vi "Window-Calibration toolbox_v6.vi"() -> ()   [LabVIEW 2017]
uses:
  Configuration code/Calibration/ToolBox/TypeDefs/Current Calibration Parameters.ctl
  Configuration code/Calibration/ToolBox/TypeDefs/ProcedureState.ctl
  Typedefs/Objective selector control enum.ctl
  <vilib>/Math Plots/3D Math Plots/3D Surface/3D Surface XCtrl/3D Surface.xctl
  <vilib>/vision/Image Controls.llb/IMAQ Image.ctl
  Configuration code/Calibration/ToolBox/TypeDefs/Procedure_State.ctl
  Configuration code/Calibration/ToolBox/TypeDefs/Control Plane.ctl
  Typedefs/HW config states enum.ctl
  Peripherals Control/XYZ Stage/Typedefs/XYZ stage data.ctl
  Peripherals Control/XYZ Stage/Typedefs/XYZ stage states.ctl
  Peripherals Control/XYZ Stage/Typedefs/XYZ channel ring.ctl
  Typedefs/Top level VI states.ctl
  Global Variables/General Globals.vi
  Configuration code/Calibration/Globals/gl_Calibration globals.vi
  Global Variables/gl_UI Ctrl Refs.vi
  <vilib>/Math Plots/3D Math Plots/3D Surface/3D Surface Datatype/Public/Plot Helper (Matrix).vi
  <resource>/objmgr/IMAQImage.rc
  <vilib>/GPower/Array/GPArray.lvlib
  Global Variables/gl_Queues.vi
  <vilib>/Math Plots/3D Math Plots/3D Surface/3D Surface Datatype/3D Surface Datatype.lvclass
  <vilib>/GPower/Array/Library/Create/Random/CreateRandomI8.vi
panel:
  in  "Plot Postion":bool
  in  "Cancel Button":bool
  in  "Record Postion":bool
  in  "Z Norm":bool
  in  "Signal Channel":enum16{"Red", "Green"}(ring)
  in  "Current Objective":T1="Olympus  20X"
  out "mini steps":dbl=100.0
  out "LL":dbl=100.0 format="%#_g µm"
  out "UL":dbl=100.0 format="%#_g µm"
  in  "miniStep size":dbl=100.0 format="%#_g µm"
  in  "Sequence":bool
  in  "Test":bool
  in  "Calibrate":bool
  in  "Tab 2":T2(tab) caption="Calibration Tab"
  in  "AOLZ":sgl(slide) scale=-200.0..200.0 scale format="%#_2f"
  in  "Y Centre":sgl(slide) caption="Y centre" scale=-1.0..1.0 scale format="%#_2f"
  in  "X Centre":sgl(slide) scale=-1.0..1.0 scale format="%#_2f"
  in  "Zero Stage":bool
  in  "XY Step Size":dbl=100.0 format="%#_g µm"
  in  "Up":bool
  in  "Left":bool
  in  "Right":bool
  in  "Down":bool
  out "Focal Plane":sgl format="Z:%#_g"
  in  "Set focal plane":bool
  in  "Z Step Size":dbl=100.0 format="%#_g µm"
  in  "Natural Plane":bool
  in  "Move Down":bool
  in  "Move Up":bool
  out "Stage XYZ Position":cluster{"X":sgl, "Y":sgl, "Z":sgl}
  in  "Current Calibration Parameters":T3
  in  "Z Angle":dbl(knob)
  in  "Y Angle":dbl(knob)
  in  "X Angle":dbl(knob) min=0.0 max=359.9 step=0.1
  in  "Sweep":enum16{"Dwell Time", "SWAT"}(ring)
  in  "Multicolumn Listbox":i32(listbox)
  out "Y Scaling":cluster{"X":dbl, "Y":dbl}[](graph)
  out "X Scaling":cluster{"X":dbl, "Y":dbl}[](graph)
  out "Z Scaling":cluster{"X":dbl, "Y":dbl}[](graph)
  in  "Reload":bool
  in  "Save config.ini":bool
  out "Z plane exec time":u32
  out "3D Surface":refnum<class "3D Plot Datatype.lvclass">[](xcontrol)
  out "Intensity Graph":i16[][](graph)
  out "Image Pixels (I16)":i16[][](array[numeric])
  out "Stage Zeroed ? 2":bool
  out "AOL Z values":i32[](array[numeric])
  out "Motor Z values":i32[](array[numeric])
  out "Stage Zeroed ?":bool
  out "Z":sgl format="Z:%#_g"
  out "Y":sgl format="Y:%#_g"
  out "X":sgl format="X:%#_g"
  out "Progress":u8(slide) scale=0.0..21.0
  out "error out":errorcluster
  out "Procedure":T4
  in  "Auto Focus":bool
  in  "Message_FrontPanel":string
  in  "Cancel":bool
  in  "Abort":bool
  in  "Next":bool
  in  "N":i32=512
  out "Stop_Ind":bool
  in  "Exit":bool
  in  "Calibration Tab":T5(tab)
  in  "Live Image intensity":cluster{i16, i16}(slide)={0, 2048} scale=0.0..4095.0
  in  "Visible(Grid)":bool
  in  "Grid Lines":u32=2 min=2 max=10 step=1
  out "Image":T6(plugin-control)
  out "Array":T6[](array[plugin-control])
  out "Analysis Graph":cluster{"X":dbl, "Y":dbl}[](graph)
  out "PSF Plot":cluster{"X":dbl, "Y":dbl}[](graph)
  out "PSF Image":T6(plugin-control)
  in  "Objectives":string(tree)
  out "Calibration.ini Path":path
  out "Calibration.ini":string
  in  "Step details":string
  in  "Step No":T7(ring)
  in  "Pockels Cell Value for pointing mode":dbl
  in  "auto-set pockel":bool
  in  "Calibration_min":dbl
  in  "Calibration_max":dbl
  in  "Search_min":dbl
  in  "Search_max":dbl
  in  "Testing Range (Norm)_max":dbl=1.0
  in  "Testing Range (Norm)_min":dbl=-1.0
  in  "Auto Calibration":bool
  in  "Measure PSF":bool
  in  "Calibration test type":T8(ring)
  in  "Calibration type":T9(ring)
  # "Current XYZ Stage Position"
  # "Natural Focal Plane Z motor position must be \nset  to Zero before using the following buttons"
  # "Calibration Options"
  # "Maximal Search Range"
  # "to"
  # "(for sums &\ndiffs only)"
  # "Calibration Range from"
  # "to"
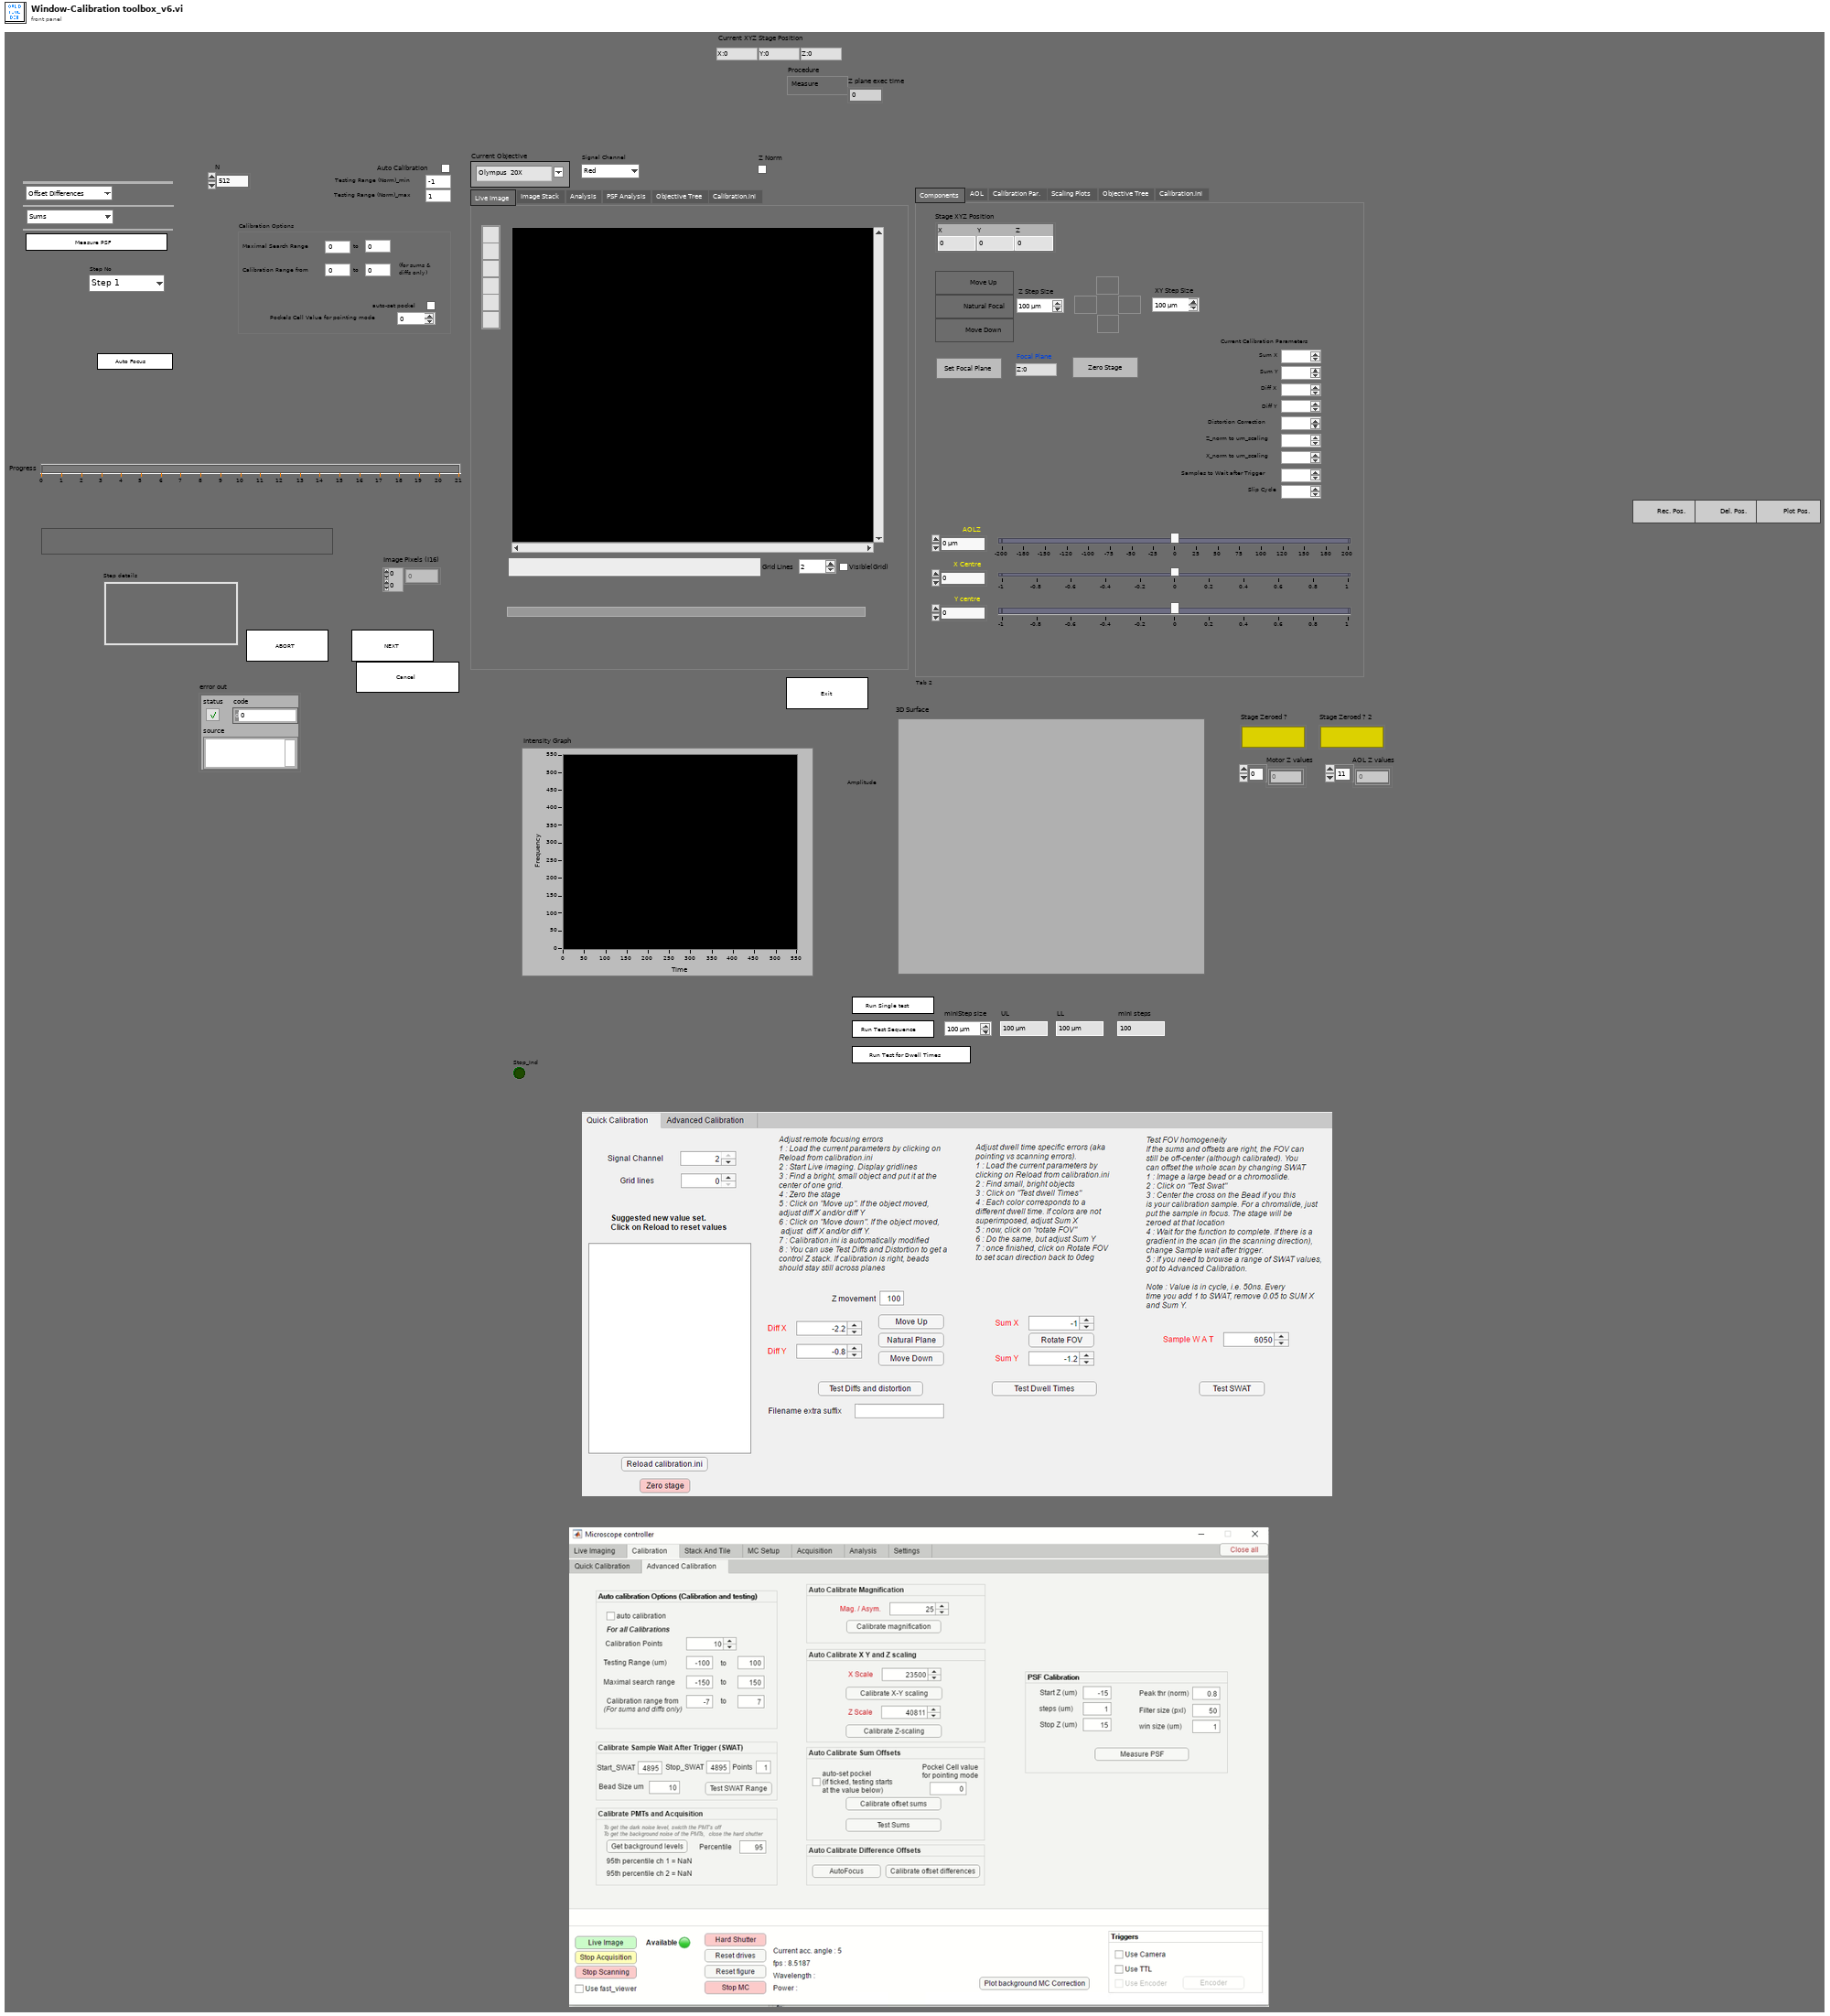
[diagram p1: front panel]
types:
  T1 = typedef "Objective selector control enum.ctl" = string
  T2 = enum32{"Components", "AOL", "Calibration Par.", "Scaling Plots", "Objective Tree", "Calibration.ini"}
  T3 = typedef "Current Calibration Parameters.ctl" = cluster{"Sum X":dbl, "Sum Y":dbl, "Diff X":dbl, "Diff Y":dbl, "Distortion Correction":dbl, "Z_norm to um_scaling":dbl, "X_norm to um_scaling":dbl, "Samples to Wait after Trigger":dbl, "Slip Cycle":dbl}
  T4 = typedef "ProcedureState.ctl" = enum16{"Measure", "Calibrate", "Sequence", "Test"}
  T5 = enum32{"Live Image", "Image Stack", "Analysis", "PSF Analysis", "Objective Tree", "Calibration.ini"}
  T6 = typedef "IMAQ Image.ctl" = refnum<image>
  T7 = enum16{"Step 1", "Step 2", "Step 3", "Step 4", "Step 5", "Step 6", "Step 7", "Step 8", "Step 9"}
  T8 = enum16{"Sums", "Diffs and Distortion", "Dwell Times"}
  T9 = enum16{"Offset Differences", "Magnification", "Offset Sums", "X-Y Scaling", "Z-Scaling"}
  T10 = enum32{"Invalid", "Standard", "Closed", "Hidden", "Minimized", "Maximized"}
  T11 = typedef "HW config states enum.ctl" = enum16{"Load from file", "Save to file", "Write all", "Read all", "Write XY stage settings", "Write DAQ FPGA settings", "Write Control FPGA settings", "Write Phys Channels", "Write System Config", "Write HW Config", "Save System Config", "Save HW Config", "Clear", "Compare from file"}
  T12 = enum8{"Enabled", "Disabled", "Disabled and Grayed Out"}
  T13 = enum16{"Initialise", "Load from file", "Save to file", "Read", "Write"}
  T14 = enum32{"Bad", "Idle", "Run top level", "Running"}
  T15 = typedef "Live graph data queue ref.ctl" = refnum<queue>
  T16 = enum32{"Image", "Image Stack", "Analysis", "PSF Analysis", "Objective Tree", "Calibration.ini"}
  T17 = typedef "Calibration config.ctl" = cluster{"Current Objective":string, "Objective Settings":T18[], "PreChirper Values Preset ?":bool, "PreChirper Settings":T19[], "PreChirper Constants":T20}
  T18 = typedef "Objective Config.ctl" = cluster{"Name":string, "Sum X":dbl, "Sum Y":dbl, "Diff X":dbl, "Diff Y":dbl, "Distortion Correction":dbl, "Z_norm to um_scaling":dbl, "X_norm to um_scaling":dbl, "Calibrated Wavelength":dbl}
  T19 = typedef "Prechirper Cal Config.ctl" = cluster{"Wavelength":i32, "Prism 1":i32, "Prism 2":i32}
  T20 = typedef "PreChirper constants.ctl" = cluster{"a 1":i32, "b 1":i32, "c 1":i32, "a 2":i32, "b 2":i32, "c 2":i32, "lmin":i32, "lmax":i32}
  T21 = typedef "System Configuration.ctl" = cluster{"Laser wavelength (nm)":dbl, "DAQ FPGA System":T22, "Control system":T23}
  T22 = typedef "DAQ FPGA system config.ctl" = cluster{"Clock Freq (MHz) ":dbl, "Samples Wait after Trigger":u16, "AOD fill":u16, "StartupDelay":i32, "Slip Cycle (clock cycles)":u32, "Add Cycle":bool}
  T23 = typedef "CTRL system config.ctl" = cluster{"AOD 1 Amplitude":i16, "AOD 2 Amplitude":i16, "AOD 3 Amplitude":i16, "AOD 4 Amplitude":i16, "AOD 5 Amplitude":i16, "AOD 6 Amplitude":i16, "T0 (ns)":dbl, "Ta (ns)":dbl, "Data Time Interval (ns)":dbl, "Ctrl FPGA Clock (MHz)":dbl}
  T24 = typedef "UI ctrl refs cluster.ctl" = cluster{"Top level VI path":path, "Top level VI ref":refnum<vi>, "User menu ref":refnum<k9>, "Sub Panel control":refnum<vi>, "Imaging Param Tab":refnum<vi>, "Occurrence-Start drivers":refnum<k4>, "Occurrence-Speed logging initialised":refnum<k4>, "Occurrence-XYZ stage initialised":refnum<k4>, "Exit button":refnum<vi>, "Status ind":refnum<vi>, "Set as origin":refnum<vi>, "Speed Logging":refnum<vi>, "Time Lapse":refnum<vi>, "Live Imaging":refnum<vi>, "AOL Z Stack":refnum<vi>, "Motor Z Stack":refnum<vi>, "Funct Acq button":refnum<vi>, "Hard Shutter":refnum<vi>, "Virtual Shutter":refnum<vi>, "Laser Power":refnum<vi>, "AOL Mode":refnum<vi>, "Frame Size":refnum<vi>, "Field of View":refnum<vi>, "Dwell Time":refnum<vi>, "Zoom":refnum<vi>, "AOL Z":refnum<vi>, "Objective":refnum<vi>, "Axis":refnum<vi>, "Paths & Names":refnum<vi>, "Experiment folder path (ind.)":refnum<vi>, "Last State (Ind.)":refnum<vi>, "Averages":refnum<vi>, "Angle (degrees)":refnum<vi>, "X centre":refnum<vi>, "Y centre":refnum<vi>, "Plane Mode":refnum<vi>, "# Planes":refnum<vi>, "Z Start":refnum<vi>, "Z Stop":refnum<vi>, "Z Step":refnum<vi>, "PMT 1":refnum<vi>, "PMT 2":refnum<vi>, "Stage XYZ Position":refnum<vi>, "Pockels@Z Start":refnum<vi>, "Pockels@Z Stop":refnum<vi>, "Obtain Z Start":refnum<vi>, "Obtain Z Stop":refnum<vi>, "Live stim.trig.period":refnum<vi>, "Live stim.trig.enable":refnum<vi>, "Movement Correction":refnum<vi>, "Load Reference Image":refnum<vi>, "XY Stage Move":refnum<vi>, "MovCor Cluster":refnum<vi>, "RefDAQParam":refnum<vi>, "Funct. Acq. Pockels Modulation":refnum<vi>, "Ref Laser Power":refnum<vi>, "Enable Video Recording":refnum<vi>, "Video Record-Live Imaging":refnum<vi>, "Video Record-Funct acq":refnum<vi>, "Reference Source":refnum<vi>, "AOL Z-stack Chirps Ready (ind)":refnum<vi>, "Target time between mov.cor. ref triggers (ms)":refnum<vi>, "Funct. Acq. Ref frame save":refnum<vi>, "Tracking button":refnum<vi>, "Show ref plots window":refnum<vi>, "Center freq ind (nm)":refnum<vi>, "Pickup mode (ind)":refnum<vi>, "Logging queue (ind)":refnum<vi>, "Back aperture power (ind.)":refnum<vi>, "Power after objective (ind.)":refnum<vi>, "Switch user":refnum<vi>, "Ls1 Conn. Status":refnum<vi>, "Ls1Tuning Status":refnum<vi>, "Ls1 Faults":refnum<vi>, "Ls1 Connection":refnum<vi>, "Ls1 Mode":refnum<vi>, "Ls1 POWER [mW]":refnum<vi>, "Ls1Shutter":refnum<vi>, "Ls1 Wavelength":refnum<vi>, "Ls1 Note":refnum<vi>, "Ls1 Confirm Wav":refnum<vi>, "Ls1 PreChrp Prism1":refnum<vi>, "Ls1 PreChrp Prism2":refnum<vi>, "Ls1 wav top Ind":refnum<vi>, "Ls1 power top Ind":refnum<vi>, "Ls1 Pump peak Hold":refnum<vi>, "Ls1 Status Ind":refnum<vi>, "Ls1 wav cancel":refnum<vi>, "Experiment Type":refnum<vi>, "Biology Information":refnum<vi>}
  T25 = typedef "AOL Z cal process refs.ctl" = cluster{"This VI":refnum<vi>, "Abort (ind)":refnum<vi>, "Next (ind)":refnum<vi>, "Cancel":refnum<vi>, "Next":refnum<vi>, "Message":refnum<vi>, "Progress":refnum<vi>}
  T26 = typedef "Image Type" = u32
  T27 = typedef "Control Plane.ctl" = enum16{"XY-X", "XY-Y", "Z"}
  T28 = typedef "Procedure_State.ctl" = cluster{"Procedure":T4, "Parameter":T27, "Symmetric":bool}
  T29 = typedef "XYZ stage states.ctl" = enum16{"Dequeue", "Initialize", "Read Position", "Read Speed Setting", "Move", "Set Max Speed", "Reset Axis", "Stop all movement"}
  T30 = typedef "XYZ channel ring.ctl" = string
  T31 = typedef "XYZ stage data.ctl" = cluster{"Command":T29, "Channel":T30, "X":sgl, "Y":sgl, "Z":sgl, "Speed":i32, "Zero":bool, "Use acknowledgement?":bool}
  T32 = typedef "Top level VI states.ctl" = enum16{"None", "Initialise UI", "<STACK PROTOCOL STATES>", "AOL Zstack-START", "AOL Zstack-STOP", "Motor Zstack-START", "Motor Zstack-STOP", "<ACQUISITION PROTOCOL STATES> ", "Functional Acquisition-START", "Functional Acquisition-STOP", "Single Plane Acquisition-START", "Single Plane Acquisition-STOP", "Volume Acquisition-START", "Volume Acquisition-STOP", "<LIVE IMAGING PROTOCOL STATES>", "Live Imaging-START", "Live Imaging-STOP", "Live Plane Imaging-START", "Live Plane Imaging-STOP", "Live Volume Imaging-START", "Live Volume Imaging-STOP", "<MOVEMENT CORRECTION PROTOCOL STATES>", "EXIT"}
  T33 = typedef "AOL_Globals.ctl" = cluster{"Imaging Protocol":T34, "Number of POI":u16, "Number of Miniscans":u16, "Number of Trials":u16, "Number of Cycles ":u64, "# Averaged Frames":u16, "Laser power (%)":u8, "Pockels (V)":dbl, "Acquisition Length (sec)":dbl, "Fill time (us)":dbl, "POI Dwell time (us)":dbl, "Miniscan Dwell time per pixel (us)":dbl, "PMT 1":dbl, "PMT 2":dbl, "Back Apperture (mA)":dbl, "Frame Size":T35, "Center Frequency":dbl, "Field of View (norm)":dbl, "DwellTime (us)":dbl, "Wavelength (nm)":dbl, "Zoom":dbl, "AOL Z":dbl, "AOL Mode":T36, "GridXY":dbl, "GridZ":dbl, "TriggerPeriod (sec)":dbl, "Number of Pixels in Miniscan":u16, "Experiment folder path":path, "X centre":dbl, "Y centre":dbl, "Angle (degrees)":dbl, "Angle Xs (degrees)":dbl, "Angle Ys (degrees)":dbl, "Plane Mode":T37, "Threshold":u16[], "Regenerate Chirps":bool, "Rectangle ROI length (pixels)":u16, "Rectangle ROI height (pixels)":u16, "AOD fill":u16, "StartupDelay":i32, "Samples Wait after Trigger":u16, "Slip Cycle":u32, "Add Cycle":bool, "Functional Mode":T38, "Z Start":dbl, "Z Stop":dbl, "# Planes":i32}
  T34 = typedef "Imaging Protocols enum.ctl" = enum16{"AOL Z-Stack", "Motor Z Stack", "Functional Acquisition", "Single Plane Acquisition", "Volume Acquisition", "Live Imaging", "Live Plane Imaging", "Live Volume Imaging"}
  T35 = typedef "Frame Size.ctl" = u16
  T36 = typedef "AOL modes.ctl" = enum16{"Raster", "Structural", "Pointing", "Mini Scan", "Alignment"}
  T37 = typedef "Plane Mode.ctl" = u16
  T38 = typedef "Functional Mode.ctl" = enum16{"Point", "Line", "Patch", "Plane", "Volume"}
  T39 = typedef "Live imaging queue element.ctl" = cluster{"Red channel":T6, "Green channel":T6, "Ref Red channel":T6, "Ref Green channel":T6, "Mov cor":bool}
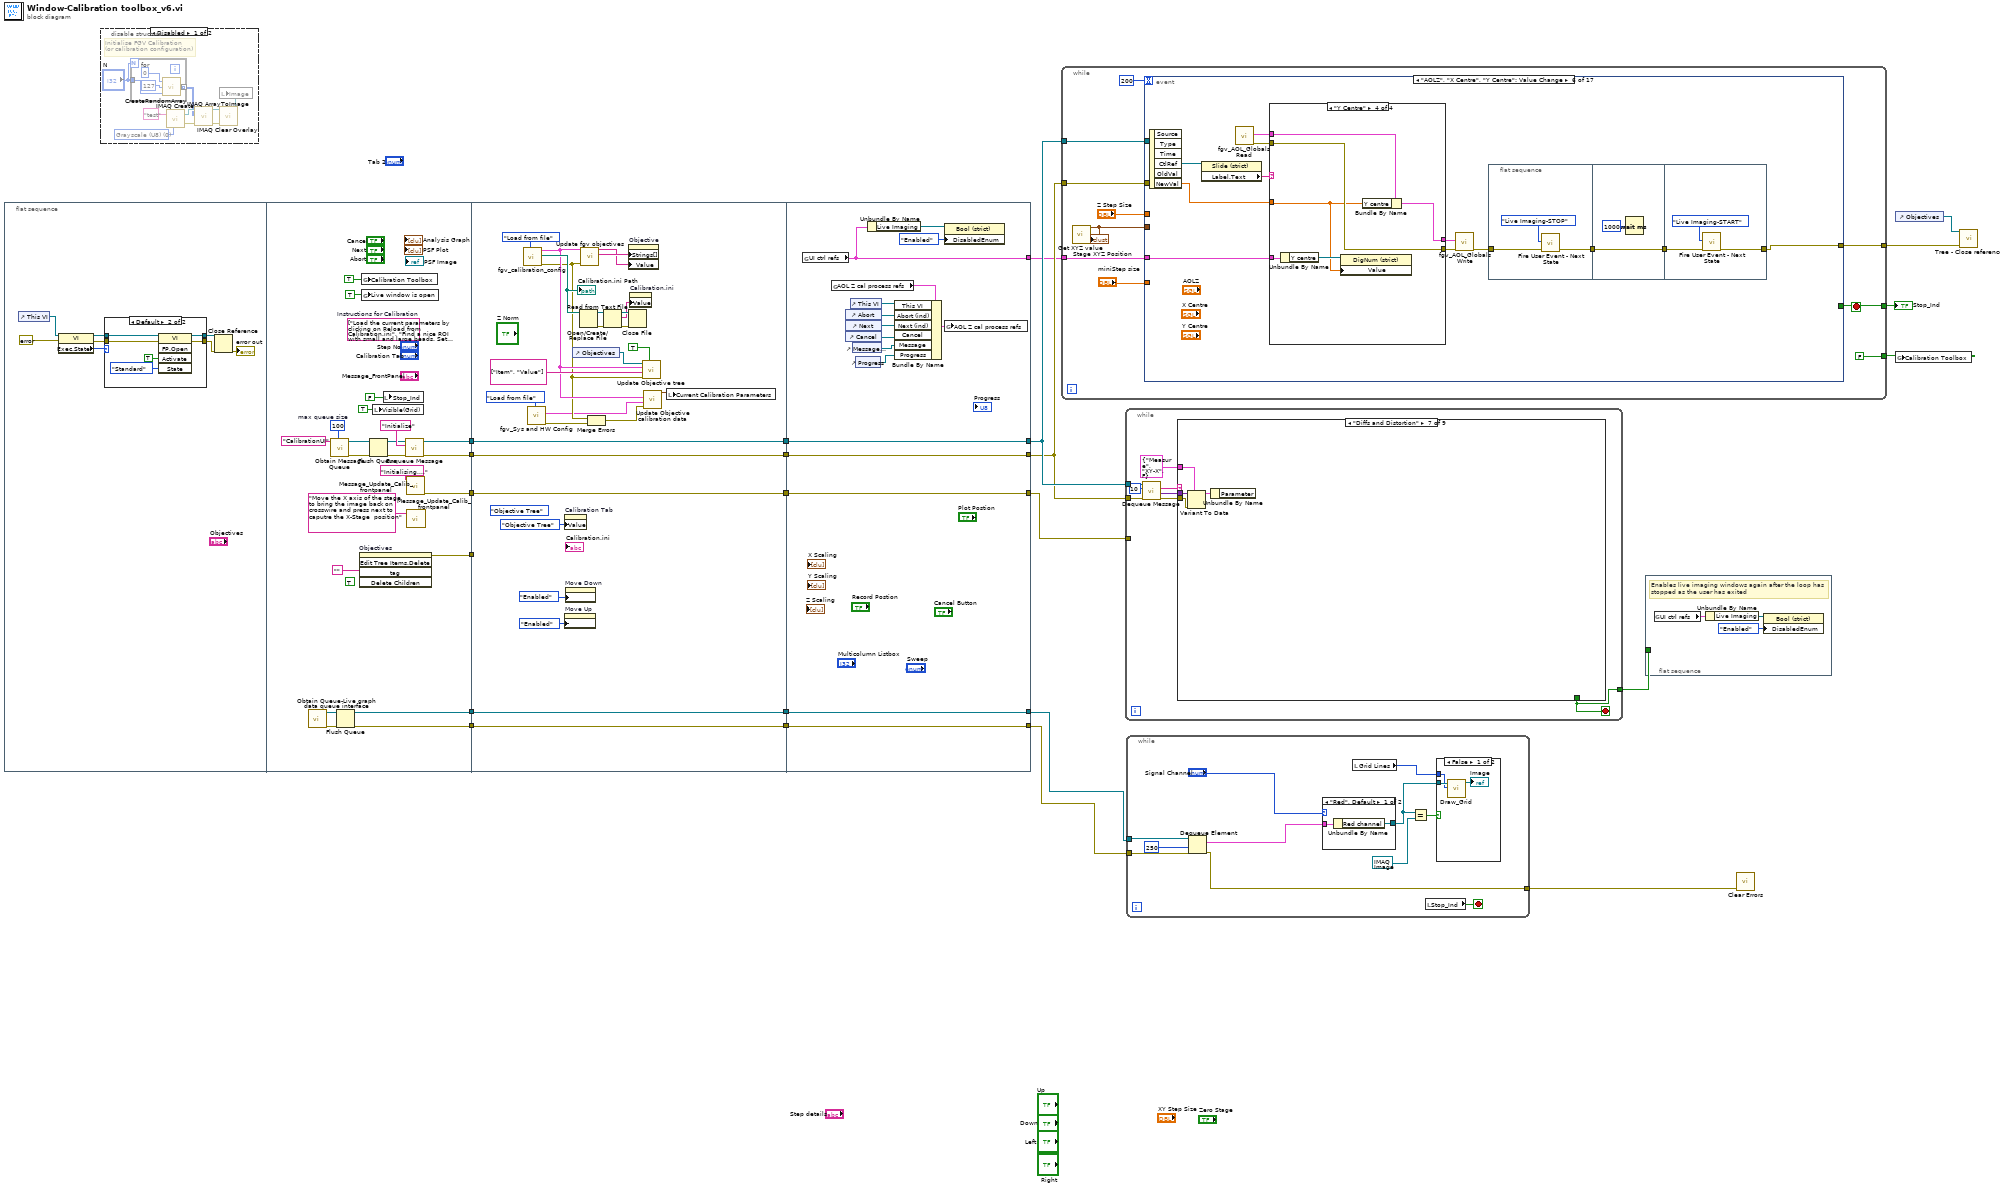
[diagram p0: block diagram]
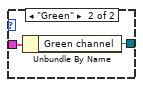
[diagram p3: hidden frame]
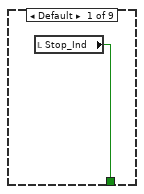
[diagram p6: hidden frame]
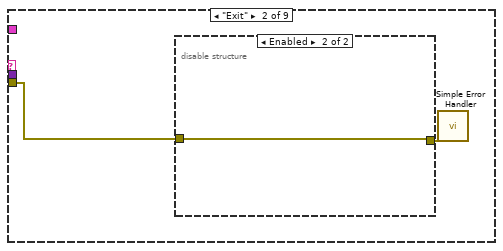
[diagram p7: hidden frame]
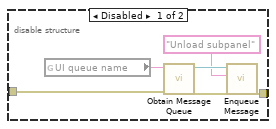
[diagram p8: hidden frame]
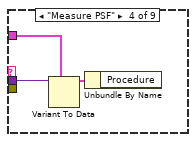
[diagram p10: hidden frame]
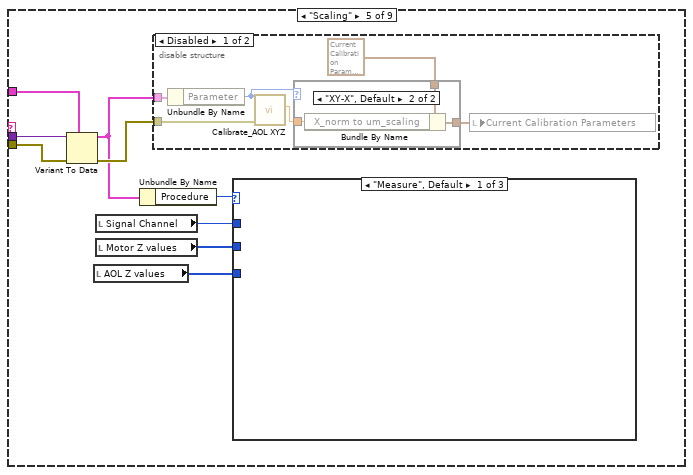
[diagram p11: hidden frame]
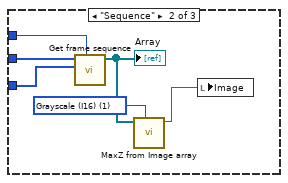
[diagram p12: hidden frame]
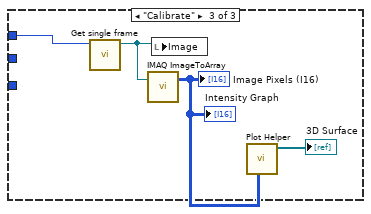
[diagram p13: hidden frame]
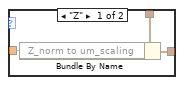
[diagram p14: hidden frame]
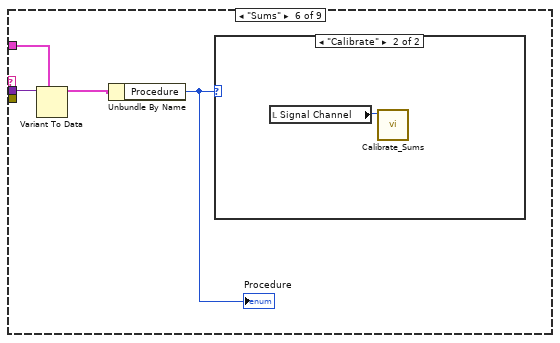
[diagram p16: hidden frame]
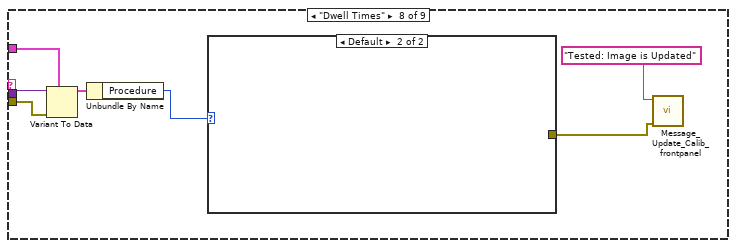
[diagram p18: hidden frame]
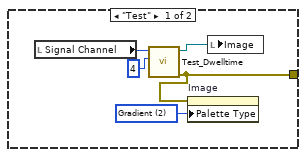
[diagram p19: hidden frame]
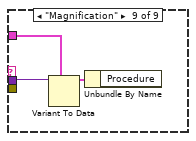
[diagram p20: hidden frame]
diagram:
  n1 = flat-sequence {
    tunnel: [w54] -> w15
    tunnel: [w53] -> w13
    tunnel: [w51] -> w11
    tunnel: [w44] -> w9
    tunnel: [w42] -> w7
    tunnel: [w41] -> w3
    tunnel: w15 -> [w88]
    tunnel: [w88] -> w14
    tunnel: w13 -> [w87]
    tunnel: [w87] -> w12
    tunnel: w11 -> [w86]
    tunnel: [w86] -> w10
    tunnel: w9 -> [w85]
    tunnel: [w85] -> w8
    tunnel: w7 -> [w84]
    tunnel: [w84] -> w6
    tunnel: w3 -> [_]
    tunnel: [w100] -> w17
    tunnel: [w101] -> w18
    tunnel: [w102] -> w19
    tunnel: [w103] -> w21
    tunnel: [w104] -> w22
    tunnel: w14 -> [w104]
    tunnel: w12 -> [w103]
    tunnel: w10 -> [w102]
    tunnel: w8 -> [w101]
    tunnel: w6 -> [w100]
    tunnel: [w92] -> w5
    frame #0 {
      n2 = control-ref of="This VI"() -> (w28:refnum<vi>)
      n3 = property class="VI"(reference=w28, error in=errorcluster {"status"=FALSE, "code"=0, "source"=""} ("error in (no error)")) -> (reference out=w27:refnum<vi>, error out=w26:errorcluster, "Exec.State"=w24:T14)
      n4 = case shown="Default" w24 {
        tunnel: [w33 w34] -> w31
        tunnel: [w32 w39] -> w30
        tunnel: w27 -> [w33 w36]
        tunnel: w26 -> [w32 w35]
        frame "Run top level" {
        }
        frame Default {
          n5 = invoke class="VI" method="FP.Open"(reference=w36, error in=w35, "Activate"=TRUE ("Activate?"), "State"=T10."Standard") -> (reference out=w34:refnum<vi>, error out=w39:errorcluster)  [unwired: 1 in, 3 out]
        }
      }
      n6 = Close Reference(reference=w31, error in (no error)=w30) -> (error out=→"error out":errorcluster)
    }
    frame #1 {
      (unwired) TRUE ("Delete Children?")
      w56 = 100  # max queue size
      (unwired) string[] ["Load the current parameters by clicking on Reload from Calibration.ini", "Find a nice ROI with small and large beads. Set PMT at 500 and adjust pockels", "Test FOV gives a sharp, single peak with Auto Focus. If yes, zero the stage. Otherwise change ROI", "Use 'Test Diffs and distortion' AND ' Test Sum' to see if the rig needs calibration for differences or sums.", "Process to teh necessary calibrations. If the performances are suboptimal, change ROI or incease laser", "If the results are bad, you can restore the previous settings by clicking on Reload from calibration.ini", "If calibration fails repetitively, try another magnification, laser pwer or FOV size.", "If calibration crashes in mid-process, go to Acquisition tab, reset drives and set the stage back to [0,0,0]. If you were in pointing mode, set teh mode toggie back to raster. Then check the pockels values."]  # Instructions for Calibration
      n7 = call "Obtain Queue-Live graph data queue interface.vi"() -> ("error out"=w45:errorcluster, "Live graphs queue"=w46:T15)  [unwired: 10 in]
      n8 = call "Obtain Message Queue.vi"("max queue size (-1, unlimited)"=w56, "Queue name"="CalibrationUI") -> ("error out"=w58:errorcluster, "Message Queue"=w60:refnum<queue>)  [unwired: 8 in]
      n9 = Flush Queue(queue=w46, error in (no error)=w45) -> (queue out=w44:T15, error out=w42:errorcluster)  [unwired: 1 out]
      n10 = invoke on="Objectives" class="Tree (strict)" method="Edit Tree Items.Delete"("tag"="") -> (error out=w41:errorcluster)  [unwired: 4 in, 4 out]
      n11 = global write "General Globals.vi" "Calibration Toolbox"(TRUE ("Calibration Toolbox")) -> ()
      n12 = global write "General Globals.vi" "Live window is open"(TRUE ("Live window is open")) -> ()
      n13 = Flush Queue(queue=w60, error in (no error)=w58) -> (queue out=w59:refnum<queue>, error out=w57:errorcluster)  [unwired: 1 out]
      n14 = local write "Visible(Grid)"(TRUE ("Visible(Grid)")) -> ()
      n15 = local write "Stop_Ind"(FALSE ("Stop_Ind")) -> ()
      n16 = call "Enqueue Message.vi"("error in (no error)"=w57, "Message"="Initialize", "Queue"=w59) -> ("error out"=w53:errorcluster, "Queue out"=w54:refnum<queue>)  [unwired: 7 in]
      n17 = call "Message_Update_Calib_frontpanel.vi"("Message"="Initialising....") -> ("error out"=w51:errorcluster)  [unwired: 10 in]
      n18 = call "Message_Update_Calib_frontpanel.vi"("Message"="Move the X axis of the stage to bring the image back on crosswire and press next to caputre the X-Stage  position") -> ()  [unwired: 10 in, 1 out]
    }
    frame #2 {
      (unwired) T16."Objective Tree" ("Calibration Tab")
      n19 = call "fgv_calibration_config.vi"("Cal config ops"=T13."Load from file") -> ("error out"=w66:errorcluster, "File Path"=w72:path, "Config cluster OUT"=w70:T17)  [unwired: 8 in]
      "Calibration.ini Path" <- w72
      n20 = call "fgv_Sys and HW Config.vi"("Function"=HW_config_states_enum."Load from file") -> ("error out"=w65:errorcluster, "System Config OUT"=w63:T21)  [unwired: 8 in, 1 out]
      n21 = property on="Calibration Tab" class="TabCtl (strict)"("Value"=T5."Objective Tree" ("Calibration Tab")) -> ()  [unwired: 2 in, 2 out]
      n22 = property on="Move Up" class="Bool"("DisabledEnum"=T12."Enabled" ("Disabled")) -> ()  [unwired: 2 in, 2 out]
      n23 = property on="Move Down" class="Bool"("DisabledEnum"=T12."Enabled" ("Disabled")) -> ()  [unwired: 2 in, 2 out]
      n24 = control-ref of="Objectives"() -> (w75:refnum<vi>)
      n25 = Open/Create/Replace File(file path (use dialog)=w72) -> (refnum out=w80:refnum<file>, error out=w79:errorcluster)  [unwired: 5 in, 1 out]
      n26 = call "Update fgv objectives.vi"("error in (no error)"=w66, "Config cluster IN"=w70) -> ("Available Objectives"=w77:string[], "Current Objective"=w76:string)  [unwired: 7 in, 1 out]
      n27 = Merge Errors(w66, w65) -> (w64:errorcluster)
      n28 = Read from Text File(file (use dialog)=w80, error in=w79) -> (refnum out=w81:refnum<file>, text=w78:string, error out=w82:errorcluster)  [unwired: 2 in, 1 out]
      n29 = property on="Objective" class="CmbBox (strict)"("Strings[]"=w77, "Value"=w76) -> ()  [unwired: 2 in, 2 out]
      n30 = Close File(refnum=w81, error in=w82) -> ()  [unwired: 2 out]
      n31 = property on="Calibration.ini" class="Str"("Value"=w78) -> ()  [unwired: 2 in, 2 out]
      n32 = call "Update Objective tree.vi"("Visible Items:Column Headers Visible"=TRUE, "error in (no error)"=w66, "Column Header Strings[]"=string[] ["Item", "Value"], "Config cluster IN"=w70, "TreeControl in"=w75) -> ()  [unwired: 6 in, 1 out]
      n33 = call "Update Objective calibration data.vi"("error in (no error)"=w64, "System Config"=w63, "Config cluster OUT"=w70) -> ("Current Calibration Parameters out"=w71:T3)  [unwired: 7 in, 1 out]
      n34 = local write "Current Calibration Parameters"(w71) -> ()
    }
    frame #3 {
      n35 = global read "gl_UI Ctrl Refs.vi" "UI ctrl refs"() -> (w92:T24)
      n36 = global read "gl_Calibration globals.vi" "AOL Z cal process refs"() -> (w94:T25)
      n37 = control-ref of="Abort"() -> (w93:refnum<vi>)
      n38 = control-ref of="Next"() -> (w99:refnum<vi>)
      n39 = control-ref of="Cancel"() -> (w95:refnum<vi>)
      n40 = control-ref of="This VI"() -> (w98:refnum<vi>)
      n41 = control-ref of="Message_FrontPanel"() -> (w96:refnum<vi>)
      n42 = control-ref of="Progress"() -> (w89:refnum<vi>)
      n43 = Unbundle By Name(w92) -> ("Live Imaging"=w91:refnum<vi>)
      n44 = Bundle By Name(cluster=w94, "This VI"=w98, "Abort (ind)"=w93, "Next (ind)"=w99, "Cancel"=w95, "Message"=w96, "Progress"=w89) -> (w97:T25)
      n45 = property class="Bool (strict)"(reference=w91, "DisabledEnum"=T12."Enabled" ("Disabled")) -> ()  [unwired: 1 in, 2 out]
      n46 = global write "gl_Calibration globals.vi" "AOL Z cal process refs"(w97) -> ()
    }
  }
  n47 = disable-structure shown="Disabled" {
    frame Disabled {
      w112 = T26 0 items=["Grayscale (U8)", "Grayscale (I16)", "Grayscale (SGL)", "Complex (CSG)", "RGB (U32)", "HSL (U32)", "RGB (U64)", "Grayscale (U16)"] ("Image Type")
      # "Initialise FGV Calibration\n(or calibration configuration)"
      n48 = for {
        N: "N" -> [_]
        tunnel: [w115] -> w109 mode=indexing
        tunnel: "N" -> [w114]
        n49 = call-poly <vilib>:"CreateRandomArray.vi"("N"=w114, "Maximum value"=i8 127, "Minimum value"=i8 0) -> ("Created array"=w115:i8[])
      }
      n50 = call "IMAQ Create"("Image Name"="test", "Image Type"=w112) -> ("New Image"=w110:T6, "error out"=w111:errorcluster)  [unwired: 3 in]
      n51 = call "IMAQ ArrayToImage"("error in (no error)"=w111, "Image Pixels (U8)"=w109, "Image"=w110) -> ("error out"=w106:errorcluster, "Image Out"=w107:T6)  [unwired: 7 in]
      n52 = call "IMAQ Clear Overlay"("error in (no error)"=w106, "Image"=w107) -> ("Image Out"=w105:T6)  [unwired: 8 in, 1 out]
      n53 = local write "Image"(w105) -> ()
    }
    frame Enabled {
    }
  }
  n54 = while {
    tunnel: [w127] -> w23
    tunnel: w22 -> [w126]
    tunnel: w21 -> [w123]
    tunnel: [FALSE ("Calibration Toolbox")] -> w20
    tunnel: w5 -> [w122]
    tunnel: [w121] -> w2
    stop <- w127 stop-if-true
    n55 = call "Get XYZ value.vi"() -> ("Stage XYZ Position"=w118:cluster{"X":sgl, "Y":sgl, "Z":sgl})  [unwired: 11 in]
    "Stage XYZ Position" <- w118
    n56 = event shown="[5] \"AOLZ\", \"X Centre\", \"Y Centre\": Value Change" {
      selector: _ -> [_ _ _ _ _ _ _ _ _ _ _ _ _ _ _ _ _]
      dyn-events: _ -> [_ _ _ _ _ _ _ _ _ _ _ _ _ _ _ _ _]
      timeout: 200 -> [_ _ _ _ _ _ _ _ _ _ _ _ _ _ _ _ _]
      tunnel: [_ TRUE _ _ _ _ _ _ _ _ _ _ _ _ _ _ _] -> w127
      tunnel: w126 -> [_ w144 _ _ _ _ _ _ w326 w380 w432 _ w455 _ _ _ _]
      tunnel: w123 -> [_ _ _ _ _ _ _ _ _ _ _ _ _ _ _ _ _]
      tunnel: w122 -> [_ _ _ w170 _ w243 w283 _ w324 w379 w422 _ _ _ _ _ _]
      tunnel: [_ _ _ _ _ w238 w278 _ _ _ _ _ _ w461 _ _ _] -> w121
      tunnel: "Z Step Size" -> [w131 _ _ w158 w237 _ _ _ _ _ _ _ _ _ _ _ _]
      tunnel: "miniStep size" -> [w130 _ _ _ w233 _ _ _ _ _ _ _ _ _ _ _ _]
      tunnel: w118 -> [w129 _ w153 w157 _ _ _ _ _ _ _ _ _ _ _ _ _]
      event Timeout {
        n57 = event-data() -> ()  [unwired: 1 in, 3 out]
        n58 = First Call?() -> (First Call?: T/F=w132:bool)
        n59 = Unbundle By Name(w129) -> ("X"=→"X":sgl, "Y"=→"Y":sgl, "Z"=w128:sgl)
        "Z" <- w128
        n60 = case shown="True" w132 {
          tunnel: w131 -> [_ w142]
          tunnel: w130 -> [_ w141]
          tunnel: w128 -> [_ w135]
          frame False {
          }
          frame True {
            n61 = Absolute Value(x=w142) -> (abs(x)=w140:dbl)
            n62 = local write "Focal Plane"(w135) -> ()
            n63 = Negate(x=w140) -> (-x=w139:dbl)
            n64 = call "Calculate Z step size.vi"("Step"=w141, "Stop"=w139, "Start"=w140) -> ("AOL Z values"=w136:dbl[], "Motor Z values"=w137:i32[], "Number of steps"=w138:i32)  [unwired: 6 in]
            n65 = local write "LL"(w139) -> ()
            n66 = local write "UL"(w140) -> ()
            n67 = local write "AOL Z values"(w136) -> ()
            n68 = local write "mini steps"(w138) -> ()
            n69 = local write "Motor Z values"(w137) -> ()
          }
        }
      }
      event Panel Close; "Exit": Value Change {
        n70 = event-data() -> ()  [unwired: 1 in, 2 out]
        n71 = case shown="True" "Exit" {
          tunnel: w144 -> [_ w151]
          frame False {
          }
          frame True {
            (unwired) enum16{"X-Y", "Z"}."X-Y" ("Parameter")
            n72 = Bundle By Name(cluster=T28 {"Procedure"=enum."Measure", "Parameter"=enum."XY-X", "Symmetric"=FALSE} ("input cluster"), "Procedure"=ProcedureState."Measure", "Parameter"=Control_Plane."XY-X") -> (w148:T28)
            n73 = call "Enqueue Message.vi"("Message Data"=w148, "Message"="Exit", "Queue"=w151) -> ()  [unwired: 7 in, 2 out]
          }
        }
      }
      event "Set focal plane": Value Change {
        n74 = event-data() -> ()  [unwired: 1 in, 6 out]
        n75 = Unbundle By Name(w153) -> ("Z"=→"Focal Plane":sgl)
      }
      event "Move Up", "Move Down", "Natural Plane": Value Change {
        n76 = event-data() -> ("CtlRef"=w173:refnum<vi>)  [unwired: 1 in, 3 out]
        n77 = Unbundle By Name(w157) -> ("Z"=w156:sgl)
        n78 = Unbundle By Name(w170) -> ("AOL Z"=w169:refnum<vi>)
        n79 = property class="Bool"(reference=w173) -> (error out=w171:errorcluster, "Label.Text"=w172:string)  [unwired: 1 in, 1 out]
        n80 = flat-sequence {
          tunnel: w172 -> [w177]
          tunnel: w171 -> [w180]
          tunnel: [w179] -> w166
          tunnel: [w178] -> w164
          tunnel: [w177] -> w162
          tunnel: [w176] -> w159
          tunnel: w158 -> [w175]
          tunnel: w156 -> [w174]
          tunnel: w166 -> [w196]
          tunnel: [w196] -> w165
          tunnel: w164 -> [w195]
          tunnel: [w195] -> w163
          tunnel: w162 -> [w194]
          tunnel: [w194] -> w161
          tunnel: [w191] -> w160
          tunnel: w159 -> [w192]
          tunnel: [w190] -> w154
          tunnel: w165 -> [w205]
          tunnel: w163 -> [w204]
          tunnel: w169 -> [w203]
          tunnel: [w202] -> w168
          tunnel: w161 -> [w202]
          tunnel: w160 -> [w201]
          tunnel: [w201] -> w167
          tunnel: [w199] -> w155
          tunnel: w154 -> [w199]
          tunnel: w168 -> [w223]
          tunnel: w167 -> [w222]
          tunnel: w155 -> [w218]
          frame #0 {
            n81 = global read "gl_Calibration globals.vi" "AOL Z cal process refs"() -> (w176:T25)
            n82 = case shown="\"Natural Plane\", Default" w177 {
              tunnel: w180 -> [_ _ _]
              tunnel: w175 -> [_ w183 w188]
              tunnel: [0.0 ("Step Size") w186 w188] -> w178
              tunnel: [w181 w184 w187] -> w179
              tunnel: w174 -> [_ w185 w189]
              frame "Natural Plane", Default {
                n83 = local read "Focal Plane"() -> (w181:sgl)
              }
              frame "Move Up" {
                n84 = Add(x=w183, y=w185) -> (x+y=w184:dbl)
                n85 = Negate(x=w183) -> (-x=w186:dbl)
              }
              frame "Move Down" {
                n86 = Subtract(x=w189, y=w188) -> (x-y=w187:dbl)
              }
            }
          }
          frame #1 {
            n87 = Unbundle By Name(w192) -> ("Message"=w191:refnum<vi>)
            n88 = disable-structure shown="Disabled" {
              frame Disabled {
                w197 = T12."Disabled and Grayed Out" ("Disabled")
                n89 = property on="Move Up" class="Bool"("DisabledEnum"=w197) -> ()  [unwired: 2 in, 2 out]
                n90 = property on="Move Down" class="Bool"("DisabledEnum"=w197) -> ()  [unwired: 2 in, 2 out]
                n91 = property on="Natural Plane" class="Bool"("DisabledEnum"=w197) -> ()  [unwired: 2 in, 2 out]
              }
              frame Enabled {
              }
            }
            n92 = property class="Str"(reference=w191, "Value"="Adjusting...") -> ()  [unwired: 1 in, 2 out]
            n93 = Tick Count (ms)() -> (millisecond timer value=w190:u32)
          }
          frame #2 {
            n94 = disable-structure shown="Enabled" {
              disable-tunnel: [w215 errorcluster {"status"=FALSE, "code"=0, "source"=""} ("error in")] -> w209
              disable-tunnel: w204 -> [w214 _]
              disable-tunnel: w203 -> [w213 _]
              frame Disabled {
                n95 = property class="Slide (strict)"(reference=w213, "Value"=w214) -> (error out=w215:errorcluster)  [unwired: 1 in, 1 out]
                n96 = call "fgv_AOL_Globals Read.vi"() -> ("AOL_Globals"=w211:T33)  [unwired: 9 in, 2 out]
                n97 = Bundle By Name(cluster=w211, "AOL Z"=w214) -> (w212:T33)
                n98 = call "fgv_AOL_Globals Write.vi"("AOL_Globals"=w212) -> ()  [unwired: 10 in, 1 out]
              }
              frame Enabled {
              }
            }
            n99 = Bundle By Name(cluster=T31 {"Command"=enum."Initialize", "Channel"="Z", "X"=0.0, "Y"=0.0, "Z"=0.0, "Speed"=0, "Zero"=FALSE, "Use acknowledgement?"=TRUE} ("XYZ Stage data to queue"), "Command"=XYZ_stage_states."Move", "Channel"=T30 "Z", "Z"=w205, "Use acknowledgement?"=FALSE) -> (w210:T31)
            n100 = call "XYZ Stage-Command request module.vi"("error in"=w209, "Command"=XYZ_stage_states."Move", "XYZ Stage data to queue"=w210) -> ()  [unwired: 4 in, 5 out]
          }
          frame #3 {
            n101 = disable-structure shown="Disabled" {
              disable-tunnel: w223 -> [w224 _]
              frame Disabled {
                n102 = case shown="\"Natural Plane\", Default" w224 {
                  frame "Move Up" {
                    n103 = property on="Move Down" class="Bool"("DisabledEnum"=T12."Enabled" ("Disabled")) -> ()  [unwired: 2 in, 2 out]
                    n104 = property on="Move Up" class="Bool"("DisabledEnum"=T12."Disabled and Grayed Out" ("Disabled")) -> ()  [unwired: 2 in, 2 out]
                  }
                  frame "Move Down" {
                    n105 = property on="Move Up" class="Bool"("DisabledEnum"=T12."Enabled" ("Disabled")) -> ()  [unwired: 2 in, 2 out]
                    n106 = property on="Move Down" class="Bool"("DisabledEnum"=T12."Disabled and Grayed Out" ("Disabled")) -> ()  [unwired: 2 in, 2 out]
                  }
                  frame "Natural Plane", Default {
                    n107 = property on="Move Up" class="Bool"("DisabledEnum"=T12."Enabled" ("Disabled")) -> ()  [unwired: 2 in, 2 out]
                    n108 = property on="Move Down" class="Bool"("DisabledEnum"=T12."Enabled" ("Disabled")) -> ()  [unwired: 2 in, 2 out]
                  }
                }
              }
              frame Enabled {
              }
            }
            n109 = Tick Count (ms)() -> (millisecond timer value=w219:u32)
            n110 = Subtract(x=w219, y=w218) -> (x-y=→"Z plane exec time":u32)
            n111 = property on="Natural Plane" class="Bool"("DisabledEnum"=T12."Enabled" ("Disabled")) -> ()  [unwired: 2 in, 2 out]
            n112 = property class="Str"(reference=w222, "Value"="Done") -> ()  [unwired: 1 in, 2 out]
          }
        }
      }
      event "Z Step Size", "miniStep size": Value Change {
        n113 = event-data() -> ()  [unwired: 1 in, 6 out]
        n114 = Absolute Value(x=w237) -> (abs(x)=w236:dbl)
        "UL" <- w236
        n115 = Negate(x=w236) -> (-x=w235:dbl)
        "LL" <- w235
        n116 = call "Calculate Z step size.vi"("Step"=w233, "Stop"=w235, "Start"=w236) -> ("AOL Z values"=→"AOL Z values":dbl[], "Motor Z values"=→"Motor Z values":i32[], "Number of steps"=→"mini steps":i32)  [unwired: 6 in]
      }
      event "AOLZ", "X Centre", "Y Centre": Value Change {
        n117 = event-data() -> ("CtlRef"=w249:refnum<vi>, "NewVal"=w242:sgl)  [unwired: 1 in, 4 out]
        n118 = property class="Slide (strict)"(reference=w249) -> ("Label.Text"=w248:string)  [unwired: 1 in, 2 out]
        n119 = call "fgv_AOL_Globals Read.vi"() -> ("error out"=w244:errorcluster, "AOL_Globals"=w247:T33)  [unwired: 9 in, 1 out]
        n120 = case shown="\"Y Centre\"" w248 {
          tunnel: w247 -> [w259 w264 w271 w277]
          tunnel: [w259 w262 w270 w275] -> w246
          tunnel: [w258 w263 w269 w276] -> w245
          tunnel: w244 -> [w258 w263 w269 w276]
          tunnel: w242 -> [_ w261 w266 w272]
          tunnel: w243 -> [_ w260 w268 w274]
          frame Default {
          }
          frame "AOLZ" {
            n121 = Unbundle By Name(w260) -> ("AOL Z"=w265:refnum<vi>)
            n122 = property class="Slide (strict)"(reference=w265, "Value"=w261) -> ()  [unwired: 1 in, 2 out]
            n123 = Bundle By Name(cluster=w264, "Y centre"=w261) -> (w262:T33)
          }
          frame "X Centre" {
            n124 = Unbundle By Name(w268) -> ("X centre"=w267:refnum<vi>)
            n125 = Bundle By Name(cluster=w271, "X centre"=w266) -> (w270:T33)
            n126 = property class="DigNum (strict)"(reference=w267, "Value"=w266) -> ()  [unwired: 1 in, 2 out]
          }
          frame "Y Centre" {
            n127 = Unbundle By Name(w274) -> ("Y centre"=w273:refnum<vi>)
            n128 = property class="DigNum (strict)"(reference=w273, "Value"=w272) -> ()  [unwired: 1 in, 2 out]
            n129 = Bundle By Name(cluster=w277, "Y centre"=w272) -> (w275:T33)
          }
        }
        n130 = call "fgv_AOL_Globals Write.vi"("error in (no error)"=w245, "AOL_Globals"=w246) -> ("error out"=w239:errorcluster)  [unwired: 9 in]
        n131 = flat-sequence {
          tunnel: w239 -> [w251]
          tunnel: [w250] -> w241
          tunnel: [w254] -> w240
          tunnel: w241 -> [w254]
          tunnel: w240 -> [w257]
          tunnel: [w256] -> w238
          frame #0 {
            n132 = call "Fire User Event - Next State.vi"("Error In"=w251, "\"UI Handler loop\" case to execute"=Top_level_VI_states."Live Imaging-STOP" ("event data / imaging mode")) -> ("Error Out"=w250:errorcluster)  [unwired: 9 in]
          }
          frame #1 {
            n133 = Wait (ms)(milliseconds to wait=u32 1000) -> ()  [unwired: 1 out]
          }
          frame #2 {
            n134 = call "Fire User Event - Next State.vi"("Error In"=w257, "\"UI Handler loop\" case to execute"=Top_level_VI_states."Live Imaging-START" ("event data / imaging mode")) -> ("Error Out"=w256:errorcluster)  [unwired: 9 in]
          }
        }
      }
      event "X Angle", "Y Angle", "Z Angle": Value Change {
        n135 = event-data() -> ("CtlRef"=w289:refnum<vi>, "NewVal"=w282:dbl)  [unwired: 1 in, 4 out]
        n136 = property class="Knob (strict)"(reference=w289) -> ("Label.Text"=w288:string)  [unwired: 1 in, 2 out]
        n137 = call "fgv_AOL_Globals Read.vi"() -> ("error out"=w287:errorcluster, "AOL_Globals"=w284:T33)  [unwired: 9 in, 1 out]
        n138 = case shown="\"Z Angle\"" w288 {
          tunnel: [w299 w300 w306 w311] -> w286
          tunnel: w287 -> [w299 w300 w306 w311]
          tunnel: [w298 w301 w305 w312] -> w285
          tunnel: w284 -> [w298 w303 w307 w313]
          tunnel: w283 -> [_ _ _ w309]
          tunnel: w282 -> [_ w302 w304 w308]
          frame Default {
          }
          frame "X Angle" {
            n139 = Bundle By Name(cluster=w303, "Angle Xs (degrees)"=w302) -> (w301:T33)
          }
          frame "Y Angle" {
            n140 = Bundle By Name(cluster=w307, "Angle Ys (degrees)"=w304) -> (w305:T33)
          }
          frame "Z Angle" {
            n141 = Unbundle By Name(w309) -> ("Angle (degrees)"=w310:refnum<vi>)
            n142 = property class="DigNum (strict)"(reference=w310, "Value"=w308) -> ()  [unwired: 1 in, 2 out]
            n143 = Bundle By Name(cluster=w313, "Angle (degrees)"=w308) -> (w312:T33)
          }
        }
        n144 = call "fgv_AOL_Globals Write.vi"("error in (no error)"=w286, "AOL_Globals"=w285) -> ("error out"=w281:errorcluster)  [unwired: 9 in]
        n145 = flat-sequence {
          tunnel: w281 -> [w291]
          tunnel: [w290] -> w279
          tunnel: [w294] -> w280
          tunnel: w279 -> [w294]
          tunnel: w280 -> [w297]
          tunnel: [w296] -> w278
          frame #0 {
            n146 = call "Fire User Event - Next State.vi"("Error In"=w291, "\"UI Handler loop\" case to execute"=Top_level_VI_states."Live Imaging-STOP" ("event data / imaging mode")) -> ("Error Out"=w290:errorcluster)  [unwired: 9 in]
          }
          frame #1 {
            n147 = Wait (ms)(milliseconds to wait=u32 100) -> ()  [unwired: 1 out]
          }
          frame #2 {
            n148 = call "Fire User Event - Next State.vi"("Error In"=w297, "\"UI Handler loop\" case to execute"=Top_level_VI_states."Live Imaging-START" ("event data / imaging mode")) -> ("Error Out"=w296:errorcluster)  [unwired: 9 in]
          }
        }
      }
      event "Save config.ini": Value Change {
        n149 = event-data() -> ()  [unwired: 1 in, 6 out]
      }
      event "Calibrate": Value Change {
        (unwired) T16."Image" ("Calibration Tab")
        n150 = event-data() -> ("NewVal"=w327:bool)  [unwired: 1 in]
        n151 = Unbundle By Name(w324) -> ("Stage XYZ Position"=w323:refnum<vi>)
        n152 = property class="Clust (strict)"(reference=w323) -> ("Value"=w322:cluster{"X":sgl, "Y":sgl, "Z":sgl})  [unwired: 1 in, 2 out]
        n153 = Unbundle By Name(w322) -> ("X"=w321:sgl, "Y"=w320:sgl, "Z"=w319:sgl)
        n154 = Equal To 0?(x=w321) -> (x = 0?=w318:bool)
        n155 = Equal To 0?(x=w320) -> (x = 0?=w317:bool)
        n156 = Equal To 0?(x=w319) -> (x = 0?=w316:bool)
        n157 = Compound Arithmetic op=AND(w318, w317, w316) -> (w315:bool)
        n158 = case shown="True" w315 {
          selector: w315 -> [_ w328]
          frame False {
          }
          frame True {
            "Stage Zeroed ?" <- w328
          }
        }
        n159 = case shown="True" w327 {
          tunnel: w326 -> [_ w331]
          tunnel: "Calibration type" -> [_ w330]
          frame False {
          }
          frame True {
            n160 = case shown="True" TRUE {
              tunnel: w331 -> [_ w340]
              tunnel: w330 -> [_ w338]
              frame False {
                n161 = One Button Dialog(message="Please move the bead to a central position and\n'zero' the XYZ stage ") -> ()  [unwired: 1 in, 1 out]
              }
              frame True {
                (unwired) enum16{"X-Y", "Z"}."X-Y" ("Parameter")
                n162 = Bundle By Name(cluster=T28 {"Procedure"=enum."Measure", "Parameter"=enum."XY-X", "Symmetric"=FALSE} ("input cluster"), "Procedure"=ProcedureState."Calibrate", "Parameter"=Control_Plane."XY-X") -> (w334:T28)
                n163 = disable-structure shown="Enabled" {
                  disable-tunnel: [w344 w368] -> w341
                  disable-tunnel: [w343 w367] -> w339
                  disable-tunnel: w338 -> [w342 _]
                  disable-tunnel: "Scaling" ("Message") -> [_ w368]
                  disable-tunnel: w334 -> [_ w367]
                  frame Disabled {
                    n164 = case shown="\"Z-Scaling\"" w342 {
                      tunnel: ["Diffs and Distortion" ("Message") "Magnification" ("Message") "Sums" ("Message") "Scaling" ("Message") "Scaling" ("Message")] -> w344
                      tunnel: [w346 w351 w355 w360 w365] -> w343
                      frame "Offset Differences", Default {
                        n165 = Bundle By Name(cluster=T28 {"Procedure"=enum."Measure", "Parameter"=enum."XY-X", "Symmetric"=FALSE} ("input cluster"), "Procedure"=ProcedureState."Calibrate") -> (w346:T28)
                      }
                      frame "Magnification" {
                        n166 = Bundle By Name(cluster=T28 {"Procedure"=enum."Measure", "Parameter"=enum."XY-X", "Symmetric"=FALSE} ("input cluster"), "Procedure"=ProcedureState."Calibrate") -> (w351:T28)
                      }
                      frame "Offset Sums" {
                        n167 = Bundle By Name(cluster=T28 {"Procedure"=enum."Measure", "Parameter"=enum."XY-X", "Symmetric"=FALSE} ("input cluster"), "Procedure"=ProcedureState."Calibrate") -> (w355:T28)
                      }
                      frame "X-Y Scaling" {
                        n168 = Bundle By Name(cluster=T28 {"Procedure"=enum."Measure", "Parameter"=enum."XY-X", "Symmetric"=FALSE} ("input cluster"), "Procedure"=ProcedureState."Calibrate", "Parameter"=enum16{"X-Y", "Z"}."X-Y") -> (w360:T28)
                      }
                      frame "Z-Scaling" {
                        n169 = Bundle By Name(cluster=T28 {"Procedure"=enum."Measure", "Parameter"=enum."XY-X", "Symmetric"=FALSE} ("input cluster"), "Procedure"=ProcedureState."Calibrate", "Parameter"=enum16{"X-Y", "Z"}."Z") -> (w365:T28)
                      }
                    }
                  }
                  frame Enabled {
                  }
                }
                n170 = call "Enqueue Message.vi"("Message Data"=w339, "Message"=w341, "Queue"=w340) -> ()  [unwired: 7 in, 2 out]
              }
            }
          }
        }
        n171 = property on="Calibration Tab" class="TabCtl (strict)"("Value"=T5."Live Image" ("Calibration Tab")) -> ()  [unwired: 2 in, 2 out]
      }
      event "Sequence": Value Change {
        (unwired) T16."Image" ("Calibration Tab")
        n172 = event-data() -> ("NewVal"=w381:bool)  [unwired: 1 in]
        n173 = Unbundle By Name(w379) -> ("Stage XYZ Position"=w378:refnum<vi>)
        n174 = property class="Clust (strict)"(reference=w378) -> ("Value"=w377:cluster{"X":sgl, "Y":sgl, "Z":sgl})  [unwired: 1 in, 2 out]
        n175 = Unbundle By Name(w377) -> ("X"=w376:sgl, "Y"=w375:sgl, "Z"=w374:sgl)
        n176 = Equal To 0?(x=w376) -> (x = 0?=w373:bool)
        n177 = Equal To 0?(x=w375) -> (x = 0?=w372:bool)
        n178 = Equal To 0?(x=w374) -> (x = 0?=w371:bool)
        n179 = Compound Arithmetic op=AND(w373, w372, w371) -> (w370:bool)
        n180 = case shown="True" w370 {
          selector: w370 -> [_ w382]
          frame False {
          }
          frame True {
            "Stage Zeroed ? 2" <- w382
          }
        }
        n181 = case shown="True" w381 {
          tunnel: w380 -> [_ w384]
          frame False {
          }
          frame True {
            n182 = case shown="True" TRUE {
              tunnel: w384 -> [_ w392]
              frame False {
                n183 = One Button Dialog(message="Please move the bead to a central position and\n'zero' the XYZ stage ") -> ()  [unwired: 1 in, 1 out]
              }
              frame True {
                (unwired) enum16{"X-Y", "Z"}."X-Y" ("Parameter")
                n184 = Bundle By Name(cluster=T28 {"Procedure"=enum."Measure", "Parameter"=enum."XY-X", "Symmetric"=FALSE} ("input cluster"), "Procedure"=ProcedureState."Sequence", "Parameter"=Control_Plane."XY-X") -> (w387:T28)
                n185 = disable-structure shown="Enabled" {
                  disable-tunnel: [w396 w420] -> w393
                  disable-tunnel: [w395 w419] -> w391
                  disable-tunnel: _ -> [w394 _]
                  disable-tunnel: "Scaling" ("Message") -> [_ w420]
                  disable-tunnel: w387 -> [_ w419]
                  frame Disabled {
                    n186 = case shown="\"Z-Scaling\"" w394 {
                      tunnel: ["Diffs and Distortion" ("Message") "Magnification" ("Message") "Sums" ("Message") "Scaling" ("Message") "Scaling" ("Message")] -> w396
                      tunnel: [w398 w403 w407 w412 w417] -> w395
                      frame "Offset Differences", Default {
                        n187 = Bundle By Name(cluster=T28 {"Procedure"=enum."Measure", "Parameter"=enum."XY-X", "Symmetric"=FALSE} ("input cluster"), "Procedure"=ProcedureState."Calibrate") -> (w398:T28)
                      }
                      frame "Magnification" {
                        n188 = Bundle By Name(cluster=T28 {"Procedure"=enum."Measure", "Parameter"=enum."XY-X", "Symmetric"=FALSE} ("input cluster"), "Procedure"=ProcedureState."Calibrate") -> (w403:T28)
                      }
                      frame "Offset Sums" {
                        n189 = Bundle By Name(cluster=T28 {"Procedure"=enum."Measure", "Parameter"=enum."XY-X", "Symmetric"=FALSE} ("input cluster"), "Procedure"=ProcedureState."Calibrate") -> (w407:T28)
                      }
                      frame "X-Y Scaling" {
                        n190 = Bundle By Name(cluster=T28 {"Procedure"=enum."Measure", "Parameter"=enum."XY-X", "Symmetric"=FALSE} ("input cluster"), "Procedure"=ProcedureState."Calibrate", "Parameter"=enum16{"X-Y", "Z"}."X-Y") -> (w412:T28)
                      }
                      frame "Z-Scaling" {
                        n191 = Bundle By Name(cluster=T28 {"Procedure"=enum."Measure", "Parameter"=enum."XY-X", "Symmetric"=FALSE} ("input cluster"), "Procedure"=ProcedureState."Calibrate", "Parameter"=enum16{"X-Y", "Z"}."Z") -> (w417:T28)
                      }
                    }
                  }
                  frame Enabled {
                  }
                }
                n192 = call "Enqueue Message.vi"("Message Data"=w391, "Message"=w393, "Queue"=w392) -> ()  [unwired: 7 in, 2 out]
              }
            }
          }
        }
        n193 = property on="Calibration Tab" class="TabCtl (strict)"("Value"=T5."Live Image" ("Calibration Tab")) -> ()  [unwired: 2 in, 2 out]
      }
      event "Test": Value Change {
        n194 = event-data() -> ("NewVal"=w433:bool)  [unwired: 1 in]
        n195 = Unbundle By Name(w422) -> ("Stage XYZ Position"=w430:refnum<vi>)
        n196 = property class="Clust (strict)"(reference=w430) -> ("Value"=w429:cluster{"X":sgl, "Y":sgl, "Z":sgl})  [unwired: 1 in, 2 out]
        n197 = Unbundle By Name(w429) -> ("X"=w428:sgl, "Y"=w427:sgl, "Z"=w426:sgl)
        n198 = Equal To 0?(x=w428) -> (x = 0?=w425:bool)
        n199 = Equal To 0?(x=w427) -> (x = 0?=w424:bool)
        n200 = Equal To 0?(x=w426) -> (x = 0?=w423:bool)
        n201 = Compound Arithmetic op=OR(w425, w424, w423) -> (w421:bool)
        n202 = case shown="True" w433 {
          tunnel: w432 -> [_ w435]
          tunnel: "Calibration test type" -> [_ w436]
          tunnel: w421 -> [_ w434]
          frame False {
          }
          frame True {
            n203 = case shown="True" w434 {
              tunnel: w436 -> [_ w439]
              tunnel: w435 -> [_ w438]
              frame False {
                n204 = One Button Dialog(message="Please move the bead to a central position and\n'zero' the XYZ stage ") -> ()  [unwired: 1 in, 1 out]
              }
              frame True {
                n205 = case shown="\"Dwell Times\"" w439 {
                  tunnel: ["Sums" ("Message") "Diffs and Distortion" ("Message") "Dwell Times" ("Message")] -> w441
                  tunnel: [w443 w448 w452] -> w440
                  frame "Sums", Default {
                    n206 = Bundle By Name(cluster=T28 {"Procedure"=enum."Measure", "Parameter"=enum."XY-X", "Symmetric"=FALSE} ("input cluster"), "Procedure"=ProcedureState."Test") -> (w443:T28)
                  }
                  frame "Diffs and Distortion" {
                    n207 = Bundle By Name(cluster=T28 {"Procedure"=enum."Measure", "Parameter"=enum."XY-X", "Symmetric"=FALSE} ("input cluster"), "Procedure"=ProcedureState."Test") -> (w448:T28)
                  }
                  frame "Dwell Times" {
                    n208 = Bundle By Name(cluster=T28 {"Procedure"=enum."Measure", "Parameter"=enum."XY-X", "Symmetric"=FALSE} ("input cluster"), "Procedure"=ProcedureState."Test") -> (w452:T28)
                  }
                }
                n209 = call "Enqueue Message.vi"("Message Data"=w440, "Message"=w441, "Queue"=w438) -> ()  [unwired: 7 in, 2 out]
              }
            }
          }
        }
      }
      event "Testing Range (Norm)_min", "Testing Range (Norm)_max", "Auto Focus", "Search_max", "Search_min", "Calibration_max", "Calibration_min", "auto-set pockel", "Pockels Cell Value for pointing mode": Value Change {
        n210 = event-data() -> ()  [unwired: 1 in, 6 out]
      }
      event "Measure PSF": Value Change {
        n211 = event-data() -> ("NewVal"=w454:bool)  [unwired: 1 in]
        n212 = case shown="True" w454 {
          tunnel: w455 -> [_ w459]
          frame False {
          }
          frame True {
            n213 = Bundle By Name(cluster=T28 {"Procedure"=enum."Measure", "Parameter"=enum."XY-X", "Symmetric"=FALSE} ("input cluster"), "Procedure"=ProcedureState."Measure") -> (w458:T28)
            n214 = call "Enqueue Message.vi"("Message Data"=w458, "Message"="Measure PSF", "Queue"=w459) -> ()  [unwired: 7 in, 2 out]
          }
        }
      }
      event "Reload": Value Change {
        n215 = event-data() -> ("NewVal"=w464:bool)  [unwired: 1 in, 5 out]
        n216 = case shown="True" w464 {
          tunnel: "Current Calibration Parameters" -> [_ w483]
          tunnel: "Current Objective" -> [_ _]
          tunnel: [errorcluster {"status"=FALSE, "code"=0, "source"=""} ("error out") w467] -> w461
          frame False {
          }
          frame True {
            (unwired) T16."Image" ("Calibration Tab")
            n217 = call "fgv_calibration_config.vi"("Cal config ops"=T13."Load from file") -> ("error out"=w472:errorcluster, "File Path"=w468:path, "Config cluster OUT"=w469:T17)  [unwired: 8 in]
            n218 = control-ref of="Objectives"() -> (w471:refnum<vi>)
            n219 = Open/Create/Replace File(file path (use dialog)=w468) -> (refnum out=w478:refnum<file>, error out=w477:errorcluster)  [unwired: 5 in, 1 out]
            n220 = property on="Calibration.ini Path" class="Path"("Value"=w468) -> ()  [unwired: 2 in, 2 out]
            n221 = call "Update fgv objectives.vi"("error in (no error)"=w472, "Config cluster IN"=w469) -> ("Available Objectives"=w476:string[], "Current Objective"=w475:string)  [unwired: 7 in, 1 out]
            n222 = Read from Text File(file (use dialog)=w478, error in=w477) -> (refnum out=w479:refnum<file>, text=w470:string, error out=w480:errorcluster)  [unwired: 2 in, 1 out]
            n223 = call "Update Objective tree.vi"("Visible Items:Column Headers Visible"=TRUE, "error in (no error)"=w472, "Column Header Strings[]"=string[] ["Item", "Value"], "Config cluster IN"=w469, "TreeControl in"=w471) -> ("error out"=w467:errorcluster)  [unwired: 6 in]
            n224 = property on="Objective" class="CmbBox (strict)"("Strings[]"=w476, "Value"=w475) -> ()  [unwired: 2 in, 2 out]
            n225 = Close File(refnum=w479, error in=w480) -> ()  [unwired: 2 out]
            n226 = property on="Calibration.ini" class="Str"("Value"=w470) -> ()  [unwired: 2 in, 2 out]
            n227 = call "Update Objective calibration data.vi"("Config cluster OUT"=w469, "Current Calibration Parameters in"=w483) -> ("Current Calibration Parameters out"=w482:T3)  [unwired: 8 in, 1 out]
            n228 = property on="Calibration Tab" class="TabCtl (strict)"("Value"=T5."Live Image" ("Calibration Tab")) -> ()  [unwired: 2 in, 2 out]
            n229 = local write "Current Calibration Parameters"(w482) -> ()
          }
        }
      }
      event Value Change {
        n230 = event-data() -> ("OldVal"=w486:T3, "NewVal"=w484:T3)  [unwired: 1 in, 4 out]
        n231 = Not Equal?(x=w486, y=w484) -> (x != y?=w485:bool)
        n232 = case shown="True" w485 {
          tunnel: w484 -> [_ w490]
          frame False {
          }
          frame True {
            n233 = call "Update_Matlab_for_calib.vi"("Current Calibration Parameters"=w490) -> ("error out"=w487:errorcluster)  [unwired: 10 in]
            n234 = flat-sequence {
              tunnel: w487 -> [w492]
              tunnel: [w491] -> w489
              tunnel: [w495] -> w488
              tunnel: w489 -> [w495]
              tunnel: w488 -> [w498]
              tunnel: [w497] -> _
              frame #0 {
                n235 = call "Fire User Event - Next State.vi"("Error In"=w492, "\"UI Handler loop\" case to execute"=Top_level_VI_states."Live Imaging-STOP" ("event data / imaging mode")) -> ("Error Out"=w491:errorcluster)  [unwired: 9 in]
              }
              frame #1 {
                n236 = Wait (ms)(milliseconds to wait=u32 1000) -> ()  [unwired: 1 out]
              }
              frame #2 {
                n237 = call "Fire User Event - Next State.vi"("Error In"=w498, "\"UI Handler loop\" case to execute"=Top_level_VI_states."Live Imaging-START" ("event data / imaging mode")) -> ("Error Out"=w497:errorcluster)  [unwired: 9 in]
              }
            }
          }
        }
      }
      event "Visible(Grid)", "Grid Lines": Value Change {
        n238 = event-data() -> ()  [unwired: 1 in, 1 out]
        n239 = case shown="True" "Visible(Grid)" {
          frame False {
            n240 = local read "Image"() -> (w501:T6)
            n241 = call "IMAQ Clear Overlay"("Image"=w501) -> ("Image Out"=w500:T6)  [unwired: 9 in, 1 out]
            n242 = local write "Image"(w500) -> ()
          }
          frame True {
            n243 = local read "Image"() -> (w508:T6)
            n244 = property class="IMAQImage"(reference=w508) -> (reference out=w505:T6, error out=w504:errorcluster, "ImageSize"=w507:cluster{"x":i32, "y":i32})  [unwired: 1 in]
            n245 = Unbundle By Name(w507) -> ("x"=w502:i32)
            n246 = Not Equal To 0?(x=w502) -> (x != 0?=w506:bool)
            n247 = case shown="True" w506 {
              tunnel: w505 -> [_ w512]
              tunnel: w504 -> [_ w511]
              tunnel: "Grid Lines" -> [_ w509]
              frame False {
              }
              frame True {
                n248 = call "Draw_Grid.vi"("error in (no error)"=w511, "Grid Lines"=w509, "Image In"=w512) -> ("Image Out"=w513:T6)  [unwired: 7 in, 1 out]
                n249 = local write "Visible(Grid)"(TRUE ("Visible(Grid)")) -> ()
                n250 = local write "Image"(w513) -> ()
              }
            }
          }
        }
      }
      event "Live Image intensity": Value Change {
        n251 = event-data() -> ("NewVal"=w515:cluster{i16, i16})  [unwired: 1 in, 5 out]
        n252 = control-ref of="Image"() -> (w514:refnum<vi>)
        n253 = call "16 bit display mapping.vi"("16 bit display mapping"=w515, "Image Display"=w514) -> ()  [unwired: 8 in, 2 out]
      }
    }
  }
  "Stop_Ind" <- w23
  n254 = while {
    tunnel: w22 -> [w523]
    tunnel: w21 -> [w519]
    tunnel: w19 -> [_]
    tunnel: [w516] -> w4
    stop <- w516 stop-if-true
    n255 = call "Dequeue Message.vi"("Error In"=w519, "timeout in ms (-1)"=10, "Message Queue"=w523) -> ("Error Out"=w518:errorcluster, "Message Data"=w521:variant, "Message"=w522:string)  [unwired: 4 in, 2 out]
    n256 = case shown="\"Diffs and Distortion\"" w522 {
      tunnel: w521 -> [_ _ _ w535 w544 w570 w574 w581 w591]
      tunnel: T28 {"Procedure"=enum."Measure", "Parameter"=enum."XY-X", "Symmetric"=FALSE} ("input cluster") -> [_ _ _ w534 w545 w569 w575 w580 w589]
      tunnel: w518 -> [_ w525 _ _ w542 _ w573 w582 _]
      tunnel: [w524 _ _ _ _ _ _ _ _] -> w516
      frame Default {
        n257 = local read "Stop_Ind"() -> (w524:bool)
      }
      frame "Exit" {
        n258 = disable-structure shown="Enabled" {
          disable-tunnel: [w529 w533] -> w526
          disable-tunnel: w525 -> [w527 w533]
          frame Disabled {
            n259 = global read "gl_Queues.vi" "UI queue name"() -> (w528:string)
            n260 = call "Obtain Message Queue.vi"("error in (no error)"=w527, "Queue name"=w528) -> ("error out"=w532:errorcluster, "Message Queue"=w531:refnum<queue>)  [unwired: 8 in]
            n261 = call "Enqueue Message.vi"("error in (no error)"=w532, "Message"="Unload subpanel", "Queue"=w531) -> ("error out"=w529:errorcluster)  [unwired: 7 in, 1 out]
          }
          frame Enabled {
          }
        }
        n262 = call <vilib>:"Simple Error Handler.vi"("error in (no error)"=w526) -> ()  [unwired: 4 in, 5 out]
      }
      frame "Initialize" {
      }
      frame "Measure PSF" {
        n263 = Variant To Data(type=w534, Variant=w535) -> (data=w536:T28)  [unwired: 1 in, 1 out]
        n264 = Unbundle By Name(w536) -> ()  [unwired: 1 out]
      }
      frame "Scaling" {
        n265 = Variant To Data(error in=w542, type=w545, Variant=w544) -> (data=w541:T28, error out=w543:errorcluster)
        n266 = local read "AOL Z values"() -> (w537:i32[])
        n267 = local read "Signal Channel"() -> (w539:enum16{"Red", "Green"})
        n268 = local read "Motor Z values"() -> (w538:i32[])
        n269 = Unbundle By Name(w541) -> ("Procedure"=w540:T4)
        n270 = disable-structure shown="Disabled" {
          disable-tunnel: w541 -> [w561 _]
          disable-tunnel: w543 -> [w560 _]
          frame Disabled {
            n271 = Unbundle By Name(w561) -> ("Parameter"=w556:T27)
            n272 = call "Calibrate_AOL XYZ.vi"("error in (no error)"=w560, "Stage Control"=w556) -> ("norm_to_um_scaling"=w557:dbl)  [unwired: 8 in, 1 out]
            n273 = case shown="\"XY-X\", Default" w556 {
              tunnel: [w564 w567] -> w559
              tunnel: T3 {"Sum X"=0.0, "Sum Y"=0.0, "Diff X"=0.0, "Diff Y"=0.0, "Distortion Correction"=0.0, "Z_norm to um_scaling"=0.0, "X_norm to um_scaling"=0.0, "Samples to Wait after Trigger"=0.0, "Slip Cycle"=0.0} ("Current Calibration Parameters") -> [w563 w566]
              tunnel: w557 -> [w562 w565]
              frame "Z" {
                n274 = Bundle By Name(cluster=w563, "Z_norm to um_scaling"=w562) -> (w564:T3)
              }
              frame "XY-X", Default {
                n275 = Bundle By Name(cluster=w566, "X_norm to um_scaling"=w565) -> (w567:T3)
              }
            }
            n276 = local write "Current Calibration Parameters"(w559) -> ()
          }
          frame Enabled {
          }
        }
        n277 = case shown="\"Measure\", Default" w540 {
          tunnel: w539 -> [_ w551 w555]
          tunnel: w538 -> [_ w550 _]
          tunnel: w537 -> [_ w549 _]
          frame "Measure", Default {
          }
          frame "Sequence" {
            w547 = T26 1 items=["Grayscale (U8)", "Grayscale (I16)", "Grayscale (SGL)", "Complex (CSG)", "RGB (U32)", "HSL (U32)", "RGB (U64)", "Grayscale (U16)"] ("Image Type")
            n278 = call "Get frame sequence.vi"("Signal Channel"=w551, "AOL Z values"=w549, "Motor Z values"=w550) -> ("Array"=w548:T6[])  [unwired: 7 in, 1 out]
            "Array" <- w548
            n279 = call "MaxZ from Image array.vi"("Image Type"=w547, "Array"=w548) -> ("Image 2"=w546:T6)  [unwired: 8 in, 1 out]
            n280 = local write "Image"(w546) -> ()
          }
          frame "Calibrate" {
            n281 = call "Get single frame.vi"("Signal Channel"=w555) -> ("Image"=w554:T6)  [unwired: 9 in, 1 out]
            n282 = call "IMAQ ImageToArray"("Image"=w554) -> ("Image Pixels (I16)"=w552:i16[][])  [unwired: 3 in, 4 out]
            "Image Pixels (I16)" <- w552
            "Intensity Graph" <- w552
            n283 = local write "Image"(w554) -> ()
            n284 = call-poly <vilib>:"Plot Helper.vi"("z matrix"=w552) -> ("3D Plot lvclass Array out"=→"3D Surface":refnum<class "3D Plot Datatype.lvclass">[])  [unwired: 5 in, 5 out]
          }
        }
      }
      frame "Sums" {
        n285 = Variant To Data(type=w569, Variant=w570) -> (data=w571:T28)  [unwired: 1 in, 1 out]
        n286 = Unbundle By Name(w571) -> ("Procedure"=w568:T4)
        "Procedure" <- w568
        n287 = case shown="\"Calibrate\"" w568 {
          frame "Test", Default {
          }
          frame "Calibrate" {
            n288 = local read "Signal Channel"() -> (w572:enum16{"Red", "Green"})
            n289 = call "Calibrate_Sums.vi"("Signal Channel"=w572) -> ()  [unwired: 8 in, 3 out]
          }
        }
      }
      frame "Diffs and Distortion" {
        n290 = Variant To Data(error in=w573, type=w575, Variant=w574) -> (data=w576:T28)  [unwired: 1 out]
        n291 = Unbundle By Name(w576) -> ()  [unwired: 1 out]
      }
      frame "Dwell Times" {
        n292 = Variant To Data(error in=w582, type=w580, Variant=w581) -> (data=w583:T28)  [unwired: 1 out]
        n293 = Unbundle By Name(w583) -> ("Procedure"=w579:T4)
        n294 = case shown="Default" w579 {
          tunnel: [w585 _] -> w578
          frame "Test" {
            w584 = u32 2 items=["Grayscale", "Binary", "Gradient", "Rainbow", "Temperature", "User Defined", "Binary 16 Bit", "Gradient 16 Bit", "Rainbow 16 Bit", "Temperature 16 Bit", "User Defined 16 Bit"] ("Palette:Palette Type")
            n295 = local read "Signal Channel"() -> (w588:enum16{"Red", "Green"})
            n296 = call "Test_Dwelltime.vi"("number of points"=4, "Signal Channel"=w588) -> ("error out"=w585:errorcluster, "MaxProj"=w587:T6)  [unwired: 8 in]
            n297 = property on="Image" class="ImageControl"(error in=w585, "Palette Type"=w584) -> ()  [unwired: 1 in, 2 out]
            n298 = local write "Image"(w587) -> ()
          }
          frame Default {
          }
        }
        n299 = call "Message_Update_Calib_frontpanel.vi"("error in (no error)"=w578, "Message"="Tested: Image is Updated") -> ()  [unwired: 9 in, 1 out]
      }
      frame "Magnification" {
        n300 = Variant To Data(type=w589, Variant=w591) -> (data=w590:T28)  [unwired: 1 in, 1 out]
        n301 = Unbundle By Name(w590) -> ()  [unwired: 1 out]
      }
    }
  }
  n302 = while {
    tunnel: w18 -> [w602]
    tunnel: w17 -> [w599]
    tunnel: [w597] -> w16
    stop <- w600 stop-if-true
    n303 = Dequeue Element(queue=w602, timeout in ms (-1)=250, error in (no error)=w599) -> (element=w601:T39, error out=w597:errorcluster)  [unwired: 2 out]
    n304 = case shown="\"Red\", Default" "Signal Channel" {
      tunnel: w601 -> [w604 w606]
      tunnel: [w603 w605] -> w595
      frame "Red", Default {
        n305 = Unbundle By Name(w604) -> ("Red channel"=w603:T6)
      }
      frame "Green" {
        n306 = Unbundle By Name(w606) -> ("Green channel"=w605:T6)
      }
    }
    n307 = local read "Grid Lines"() -> (w592:u32)
    n308 = Equal?(x=w595, y=T6 refnum) -> (x = y?=w593:bool)
    n309 = local read "Stop_Ind"() -> (w600:bool)
    n310 = case shown="False" w593 {
      tunnel: w595 -> [w609 _]
      tunnel: w592 -> [w607 _]
      frame False {
        n311 = call "Draw_Grid.vi"("Grid Lines"=w607, "Image In"=w609) -> ("Image Out"=→"Image":T6)  [unwired: 8 in, 1 out]
      }
      frame True {
      }
    }
  }
  n312 = flat-sequence {
    tunnel: w4 -> [_]
    frame #0 {
      # "Enables live imaging windows again after the loop has stopped as the user has exited"
      n313 = global read "gl_UI Ctrl Refs.vi" "UI ctrl refs"() -> (w612:T24)
      n314 = Unbundle By Name(w612) -> ("Live Imaging"=w611:refnum<vi>)
      n315 = property class="Bool (strict)"(reference=w611, "DisabledEnum"=T12."Enabled" ("Disabled")) -> ()  [unwired: 1 in, 2 out]
    }
  }
  n316 = call <vilib>:"Clear Errors.vi"("error in (no error)"=w16) -> ()  [unwired: 5 in, 2 out]
  n317 = control-ref of="Objectives"() -> (w1:refnum<vi>)
  n318 = global write "General Globals.vi" "Calibration Toolbox"(w20) -> ()
  n319 = call "Tree - Close reference.vi"("error in (no error)"=w2, "TreeControl in"=w1) -> ()  [unwired: 9 in, 1 out]
